vi "week4_timer_LV17.vi"() -> ()   [LabVIEW 2017]
panel:
  out "Waveform Chart":dbl(graph)
  out "Boolean":bool
  out "Progress bar":u8(slide) scale=0.0..10.0
  out "Operation":bool
  out "Timer count-down [seconds]":dbl format="%.3g"
  in  "Time to wait [seconds]":dbl
  in  "stop":bool
  # "A"
  # "B"
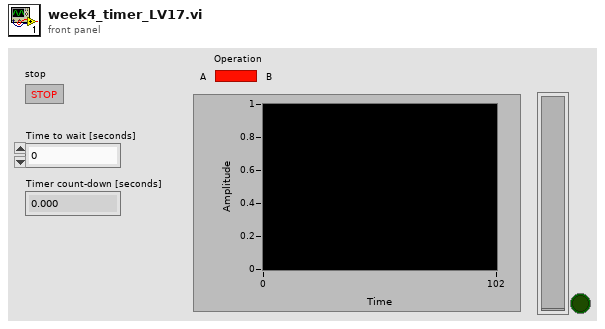
[diagram p1: front panel]
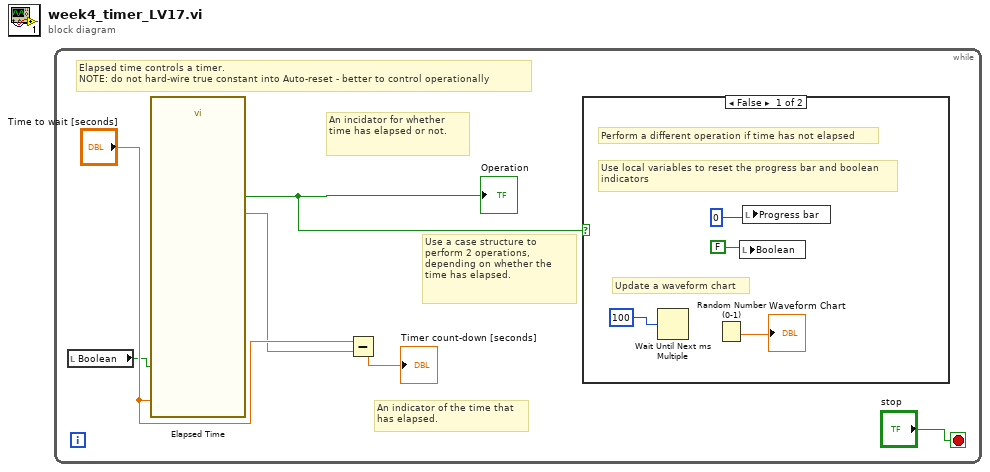
[diagram p0: block diagram]
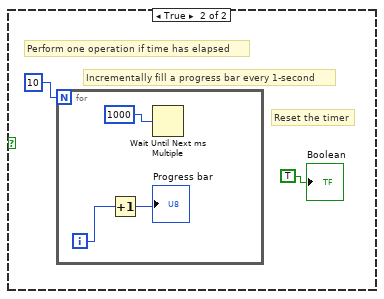
[diagram p2: hidden frame]
diagram:
  n1 = while {
    stop <- "stop" stop-if-true
    # "Use a case structure to perform 2 operations, \ndepending on whether the time has elapsed."
    # "An incidator for whether time has elapsed or not."
    # "An indicator of the time that\nhas elapsed."
    # "Elapsed time controls a timer. \nNOTE: do not hard-wire true constant into Auto-reset - better to control operationally"
    n2 = local read "Boolean"() -> (w1:bool)
    n3 = call "Elapsed Time"("Time Target (s)"="Time to wait [seconds]", "Reset"=w1) -> ("Elapsed Time (s)"=w4:dbl, "Time has Elapsed"=w2:bool)  [unwired: 10 in, 6 out]
    "Operation" <- w2
    n4 = Subtract(x="Time to wait [seconds]", y=w4) -> (x-y=→"Timer count-down [seconds]":dbl)
    n5 = case shown="False" w2 {
      frame False {
        # "Update a waveform chart"
        # "Use local variables to reset the progress bar and boolean\nindicators"
        # "Perform a different operation if time has not elapsed"
        n6 = Wait Until Next ms Multiple(millisecond multiple=100) -> ()  [unwired: 1 out]
        n7 = Random Number (0-1)() -> (number: 0 to 1=→"Waveform Chart":dbl)
        n8 = local write "Boolean"(FALSE) -> ()
        n9 = local write "Progress bar"(0) -> ()
      }
      frame True {
        # "Reset the timer"
        # "Incrementally fill a progress bar every 1-second"
        # "Perform one operation if time has elapsed"
        n10 = for {
          N: 10 -> [_]
          i -> [w13]
          n11 = Increment(x=w13) -> (x+1=→"Progress bar":i32)
          n12 = Wait Until Next ms Multiple(millisecond multiple=1000) -> ()  [unwired: 1 out]
        }
        "Boolean" <- TRUE
      }
    }
  }
